vi "Organize Folders.vi"() -> ()   [LabVIEW 2024]
uses:
  <userlib>/_OpenG.lib/file/file.llb/Strip Path Extension - String__ogtk.vi
  <userlib>/_OpenG.lib/file/file.llb/openg_file.lvlib
panel:
  in  "clear filter":bool
  in  "move":bool
  in  "Series Data":i32(listbox)
  in  "Filter":string
  in  "Series Folders":i32(listbox)
  in  "Stop":bool
  in  "Top Folders":i32(listbox)
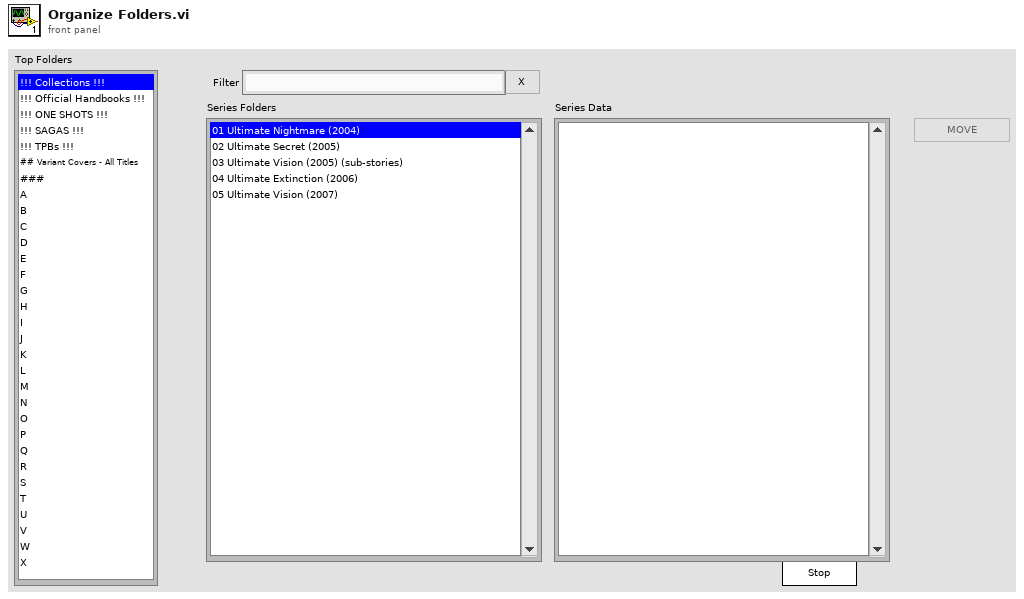
[diagram p1: front panel]
types:
  T1 = enum32{"Invalid", "Standard", "Closed", "Hidden", "Minimized", "Maximized"}
  T2 = enum32{"invalid app kind", "Development System", "Run Time System", "Student Edition", "Embedded LabVIEW", "Evaluation", "Custom"}
  T3 = enum8{"Enabled", "Disabled", "Disabled and Grayed Out"}
  T4 = cluster{"Core":cluster{"Current VI Reference":refnum<vi>, "Close Panel on Exit?":bool}, "parent path":path, "series folders":string[], "data.series path":path, "series data":string[], "old series path":path, "new series path":path}
  T5 = cluster{"Current VI Reference":refnum<vi>, "Close Panel on Exit?":bool}
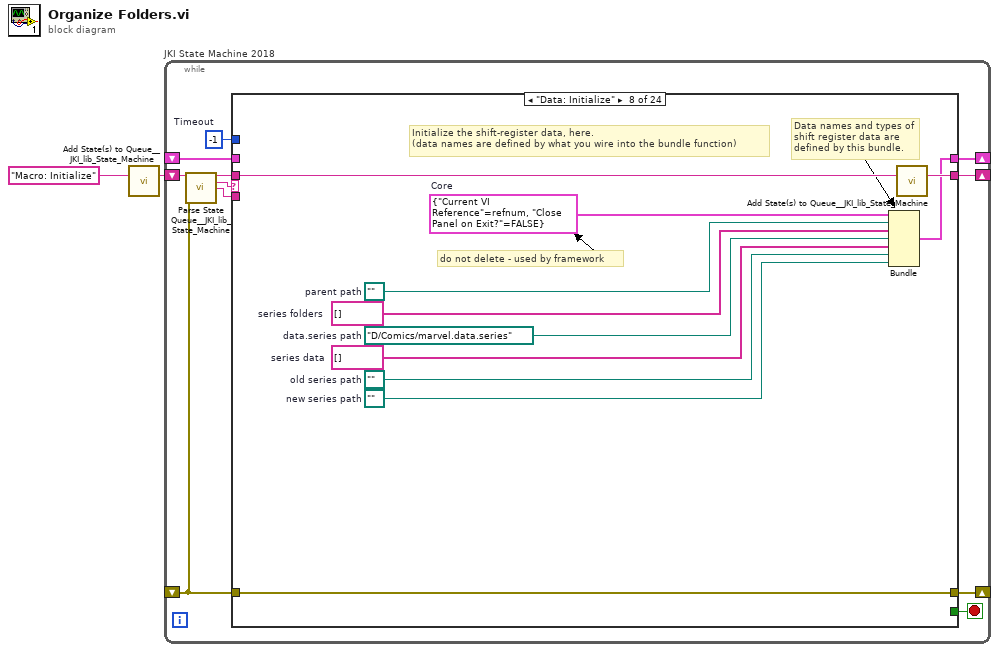
[diagram p0: block diagram]
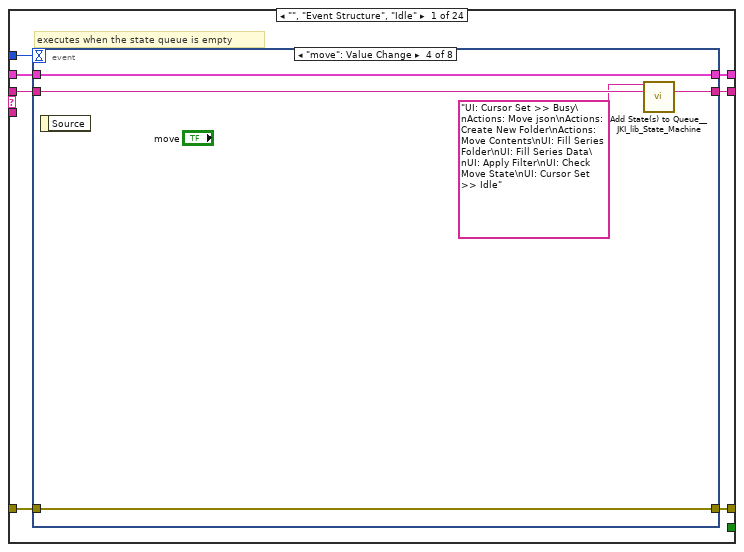
[diagram p2: hidden frame]
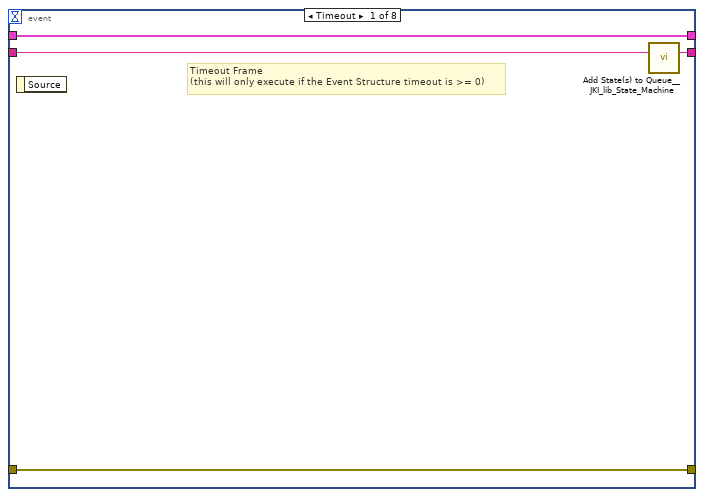
[diagram p3: hidden frame]
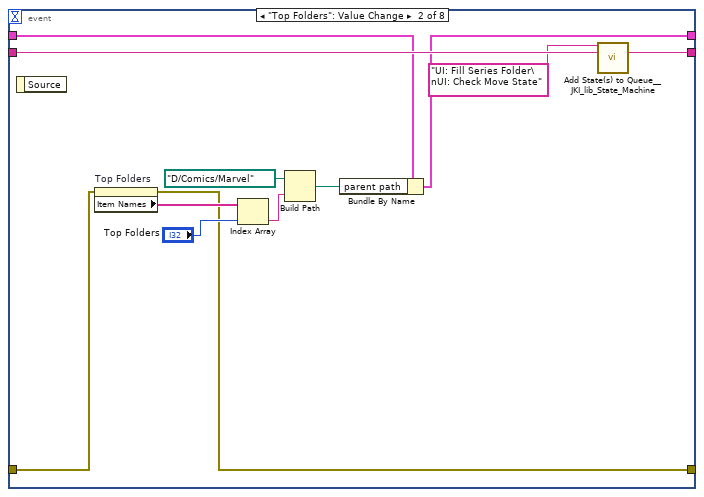
[diagram p4: hidden frame]
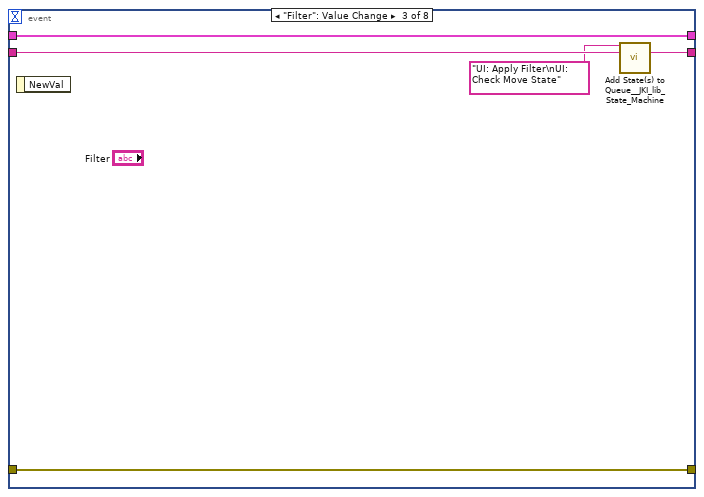
[diagram p5: hidden frame]
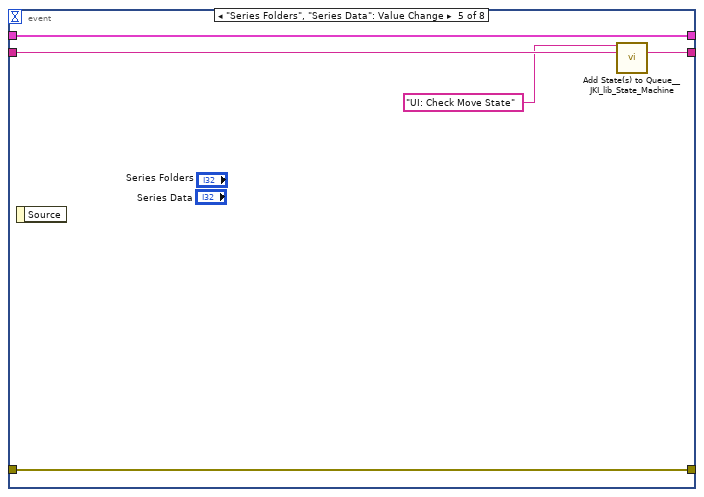
[diagram p6: hidden frame]
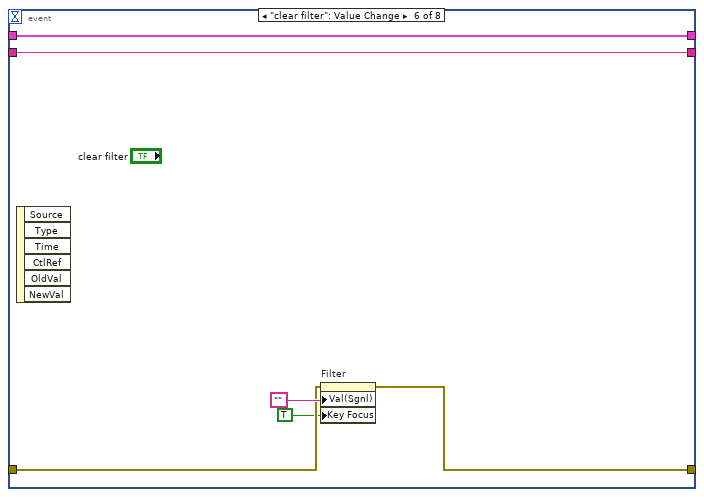
[diagram p7: hidden frame]
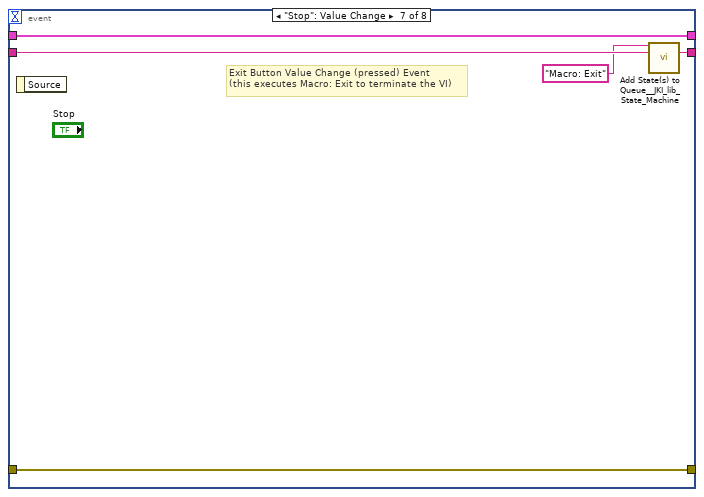
[diagram p8: hidden frame]
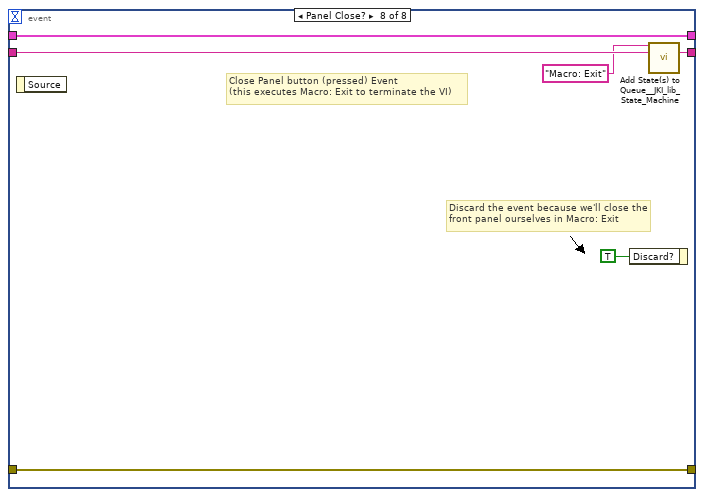
[diagram p9: hidden frame]
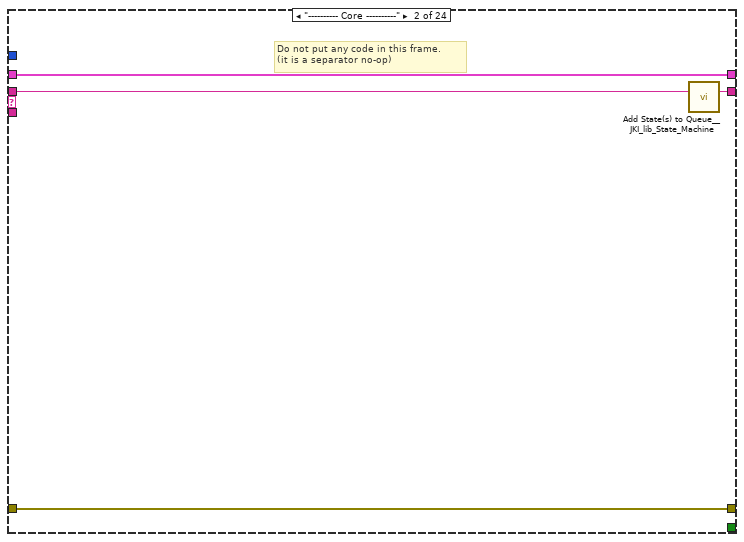
[diagram p10: hidden frame]
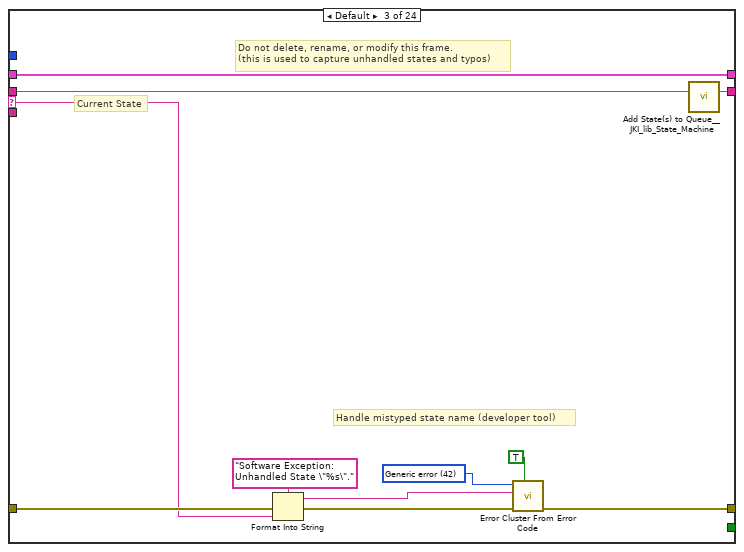
[diagram p11: hidden frame]
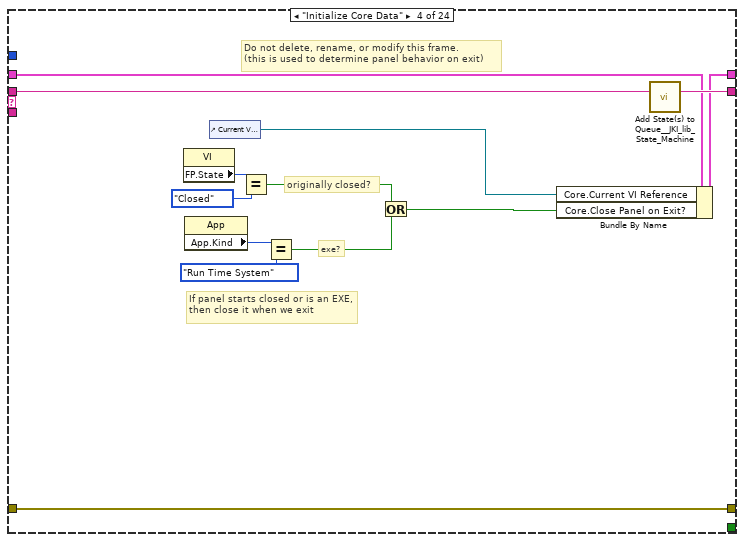
[diagram p12: hidden frame]
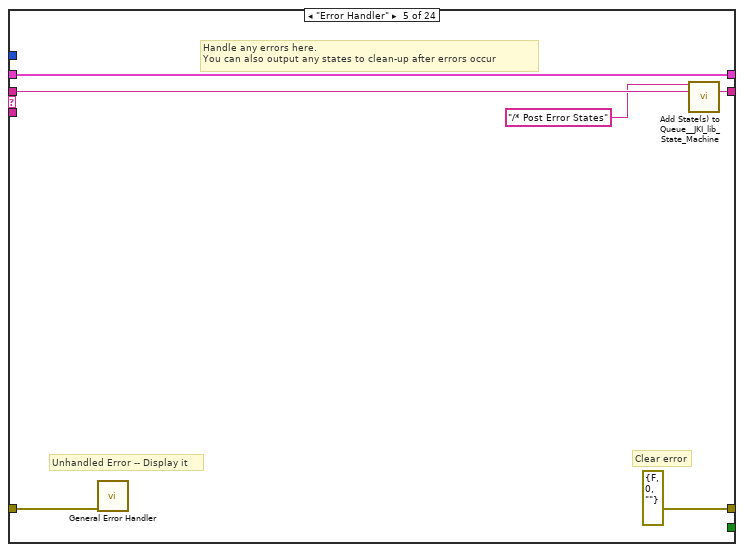
[diagram p13: hidden frame]
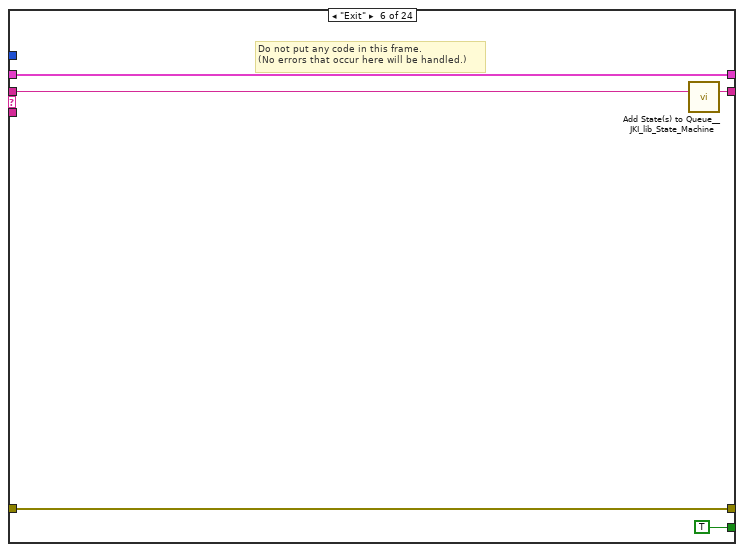
[diagram p14: hidden frame]
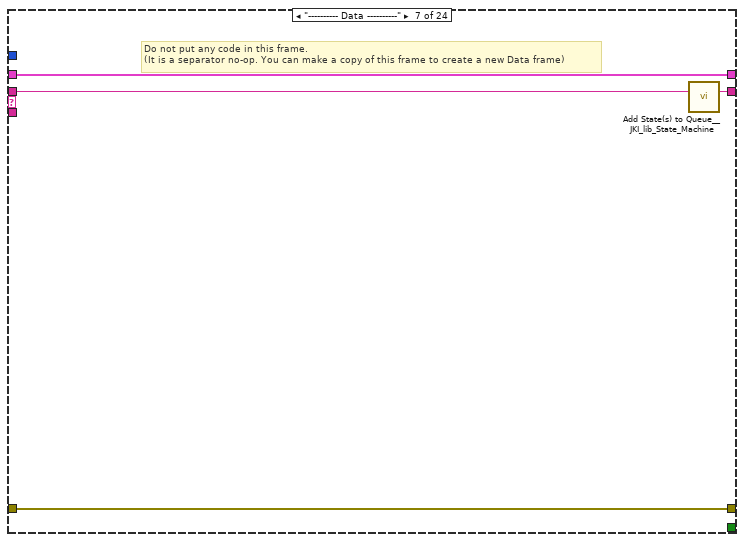
[diagram p15: hidden frame]
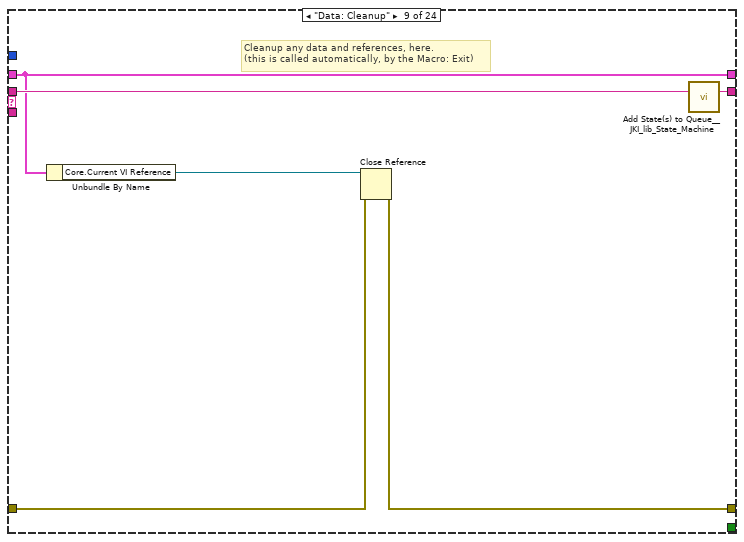
[diagram p16: hidden frame]
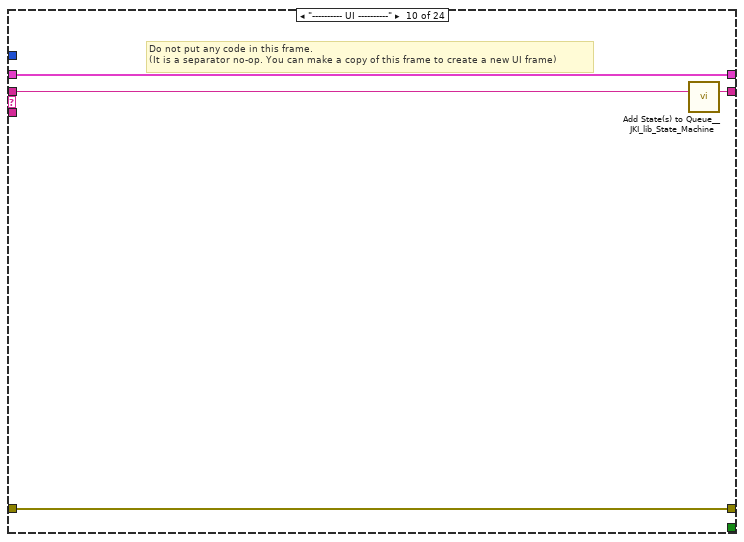
[diagram p17: hidden frame]
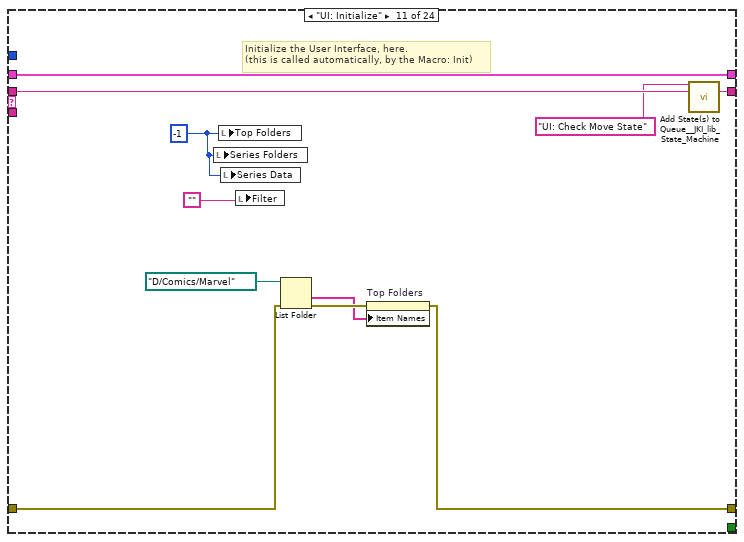
[diagram p18: hidden frame]
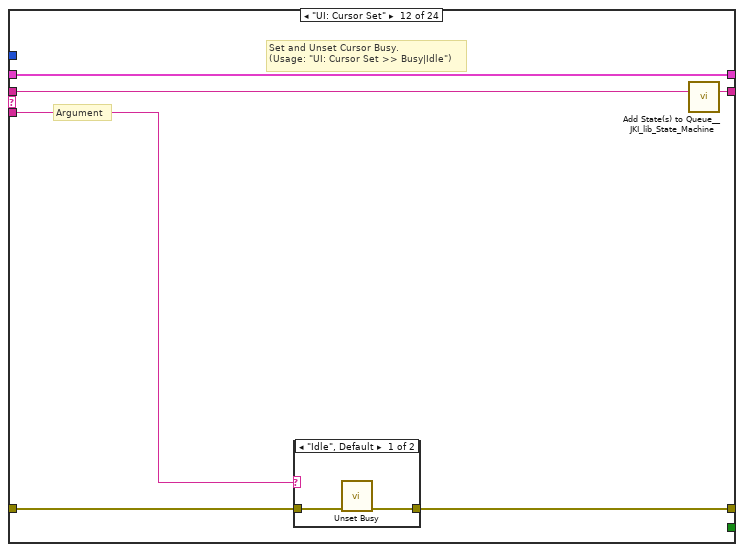
[diagram p19: hidden frame]
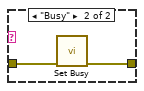
[diagram p20: hidden frame]
diagram:
  n1 = call <vilib>:"Add State(s) to Queue__JKI_lib_State_Machine.vi"("State(s) in (\"\")"="Macro: Initialize") -> ("States Out"=w2:string)  [unwired: 14 in]
  n2 = while "JKI State Machine 2018" {
    shift-right: [w6] -> _
    shift-left: _ -> [w5]
    shift-right: [w9] -> _
    shift-left: _ -> [w3]
    shift-right: [w8] -> _
    shift-left: w2 -> [w10]
    stop <- w7 stop-if-true
    w4 = -1  # Timeout
    n3 = call <vilib>:"Parse State Queue__JKI_lib_State_Machine.vi"("State Queue"=w10, "Error In (no error)"=w3) -> ("Remaining States"=w12:string, "Current State"=w13:string, "Arguments"=w11:string)  [unwired: 11 in]
    n4 = case shown="\"Data: Initialize\"" w13 {
      selector: w13 -> [_ _ w73 _ _ _ _ _ _ _ _ _ _ _ _ _ _ _ _ _ _ _ _ _]
      tunnel: w12 -> [w20 w72 w77 w96 w102 w107 w111 w122 w128 w132 w143 w149 w160 w234 w247 w259 w280 w285 w290 w300 w304 w323 w329 w337]
      tunnel: w11 -> [_ _ _ _ _ _ _ _ _ _ _ w144 w154 _ _ _ _ _ _ _ _ _ _ _]
      tunnel: w5 -> [w18 w69 w75 w89 w99 w105 w108 _ w123 w129 w141 w147 w156 w229 w242 w258 w281 w282 w287 w297 w301 w313 w327 w335]
      tunnel: [w17 w70 w79 w93 errorcluster {"status"=FALSE, "code"=0, "source"=""} ("error out") w104 w109 w119 w124 w130 w136 w145 w157 w230 w243 w252 w271 w283 w288 w298 w302 w316 w325 w333] -> w9
      tunnel: w3 -> [w16 w70 w78 w93 w98 w104 w109 w119 w125 w130 w137 w146 w158 w232 w245 w249 w270 w283 w288 w298 w302 w315 w324 w334]
      tunnel: [w19 w71 w76 w95 w101 w106 w110 w121 w127 w131 w142 w148 w159 w234 w247 w259 w280 w284 w289 w299 w303 w322 w328 w336] -> w8
      tunnel: [_ _ _ _ _ TRUE _ _ _ _ _ _ _ _ _ _ _ _ _ _ _ _ _ _] -> w7
      tunnel: [w15 w69 w75 w94 w99 w105 w108 w120 w123 w129 w141 w147 w156 w228 w241 w258 w281 w282 w287 w297 w301 w307 w327 w335] -> w6
      tunnel: w4 -> [w14 _ _ _ _ _ _ _ _ _ _ _ _ _ _ _ _ _ _ _ _ _ _ _]
      frame "", "Event Structure", "Idle" {
        # "executes when the state queue is empty"
        n5 = event shown="[3] \"move\": Value Change" {
          selector: _ -> [_ _ _ _ _ _ _ _]
          dyn-events: _ -> [_ _ _ _ _ _ _ _]
          timeout: w14 -> [_ _ _ _ _ _ _ _]
          tunnel: w20 -> [w24 w36 w40 w45 w50 w56 w62 w68]
          tunnel: [w23 w35 w39 w44 w49 w56 w61 w67] -> w19
          tunnel: w18 -> [w21 w29 w41 w46 w51 w57 w59 w65]
          tunnel: [w22 w25 w37 w42 w47 w52 w60 w66] -> w17
          tunnel: w16 -> [w22 w26 w37 w42 w47 w54 w60 w66]
          tunnel: [w21 w27 w41 w46 w51 w57 w59 w65] -> w15
          event Timeout {
            # "Timeout Frame\n(this will only execute if the Event Structure timeout is >= 0)"
            n6 = event-data() -> ()  [unwired: 1 in, 1 out]
            n7 = call <vilib>:"Add State(s) to Queue__JKI_lib_State_Machine.vi"("State(s) in (\"\")"=w24) -> ("States Out"=w23:string)  [unwired: 14 in]
          }
          event "Top Folders": Value Change {
            n8 = event-data() -> ()  [unwired: 1 in, 1 out]
            n9 = property on="Top Folders" class="LstBox (strict)"(error in=w26) -> (error out=w25:errorcluster, "Item Names"=w32:string[])  [unwired: 1 in, 1 out]
            n10 = Index Array(array=w32, index="Top Folders") -> (element=w30:string)
            n11 = Build Path(base path=path "D:/Comics/Marvel", name or relative path=w30) -> (appended path=w28:path)
            n12 = Bundle By Name(cluster=w29, "parent path"=w28) -> (w27:T4)
            n13 = call <vilib>:"Add State(s) to Queue__JKI_lib_State_Machine.vi"("State(s) in Front (\"\")"="UI: Fill Series Folder\nUI: Check Move State" ("State(s) in Front (\"\")"), "State(s) in (\"\")"=w36) -> ("States Out"=w35:string)  [unwired: 13 in]
          }
          event "Filter": Value Change {
            n14 = event-data() -> ()  [unwired: 1 in, 1 out]
            n15 = call <vilib>:"Add State(s) to Queue__JKI_lib_State_Machine.vi"("State(s) in Front (\"\")"="UI: Apply Filter\nUI: Check Move State" ("State(s) in Front (\"\")"), "State(s) in (\"\")"=w40) -> ("States Out"=w39:string)  [unwired: 13 in]
          }
          event "move": Value Change {
            n16 = event-data() -> ()  [unwired: 1 in, 1 out]
            n17 = call <vilib>:"Add State(s) to Queue__JKI_lib_State_Machine.vi"("State(s) in Front (\"\")"="UI: Cursor Set >> Busy\nActions: Move json\nActions: Create New Folder\nActions: Move Contents\nUI: Fill Series Folder\nUI: Fill Series Data\nUI: Apply Filter\nUI: Check Move State\nUI: Cursor Set >> Idle" ("State(s) in Front (\"\")"), "State(s) in (\"\")"=w45) -> ("States Out"=w44:string)  [unwired: 13 in]
          }
          event "Series Folders", "Series Data": Value Change {
            n18 = event-data() -> ()  [unwired: 1 in, 1 out]
            n19 = call <vilib>:"Add State(s) to Queue__JKI_lib_State_Machine.vi"("State(s) in Front (\"\")"="UI: Check Move State" ("State(s) in Front (\"\")"), "State(s) in (\"\")"=w50) -> ("States Out"=w49:string)  [unwired: 13 in]
          }
          event "clear filter": Value Change {
            n20 = event-data() -> ()  [unwired: 1 in, 6 out]
            n21 = property on="Filter" class="Str"(error in=w54, "Val(Sgnl)"="", "Key Focus"=TRUE) -> (error out=w52:errorcluster)  [unwired: 1 in, 1 out]
          }
          event "Stop": Value Change {
            # "Exit Button Value Change (pressed) Event\n(this executes Macro: Exit to terminate the VI)"
            n22 = event-data() -> ()  [unwired: 1 in, 1 out]
            n23 = call <vilib>:"Add State(s) to Queue__JKI_lib_State_Machine.vi"("State(s) in Front (\"\")"="Macro: Exit", "State(s) in (\"\")"=w62) -> ("States Out"=w61:string)  [unwired: 13 in]
          }
          event Panel Close? {
            # "Discard the event because we'll close the front panel ourselves in Macro: Exit"
            # "Close Panel button (pressed) Event\n(this executes Macro: Exit to terminate the VI)"
            n24 = event-data() -> ()  [unwired: 1 in, 1 out]
            n25 = event-data("Discard?"=TRUE) -> ()  [unwired: 1 in, 1 out]
            n26 = call <vilib>:"Add State(s) to Queue__JKI_lib_State_Machine.vi"("State(s) in Front (\"\")"="Macro: Exit", "State(s) in (\"\")"=w68) -> ("States Out"=w67:string)  [unwired: 13 in]
          }
        }
      }
      frame "---------- Core ----------" {
        # "Do not put any code in this frame.\n(it is a separator no-op)"
        n27 = call <vilib>:"Add State(s) to Queue__JKI_lib_State_Machine.vi"("State(s) in (\"\")"=w72) -> ("States Out"=w71:string)  [unwired: 14 in]
      }
      frame Default {
        w82 = 42 items=["No error", "Argument error", "Memory is full", "Out of zone", "End of file", "File already open", "Generic file I/O error", "File not found", "File permission error", "Disk is full", "Duplicate path", "Too many files open", "System feature not enabled", "Resource file not found", "Cannot add resource", "Resource not found", "Image not found", "Image memory error", "Pen does not exist", "Config type invalid", "Config token not found", "Config parse error", "Config memory error", "Bad external code format", "Bad external code offset", "External code not present", "Null window", "Destroy window error", "Null menu", "Print aborted", "Bad print record", "Print driver error", "Windows error during printing", "Memory error during printing", "Print dialog error", "Generic print error", "Invalid device refnum", "Device not found", "Device parameter error", "Device unit error", "Cannot open device", "Device call aborted", "Generic error", "Cancelled by user", "Object ID too low", "Object ID too high", "Object not in heap", "Unknown heap", "Unknown object (invalid DefProc)", "Unknown object (DefProc not in table)", "Message out of range", "Invalid (null) method", "Unknown message", "Manager call not supported", "Bad address", "Network operation in progress", "Network operation timed out", "Connection is busy", "Network attribute not supported", "Network error", "Address in use", "System out of memory", "Connection aborted", "Connection refused", "Not connected", "Already connected", "Connection closed", "Initialization error (interapplication manager)", "Bad occurrence", "Wait on unbound occurrence handler", "Occurrence queue overflow", "Datalog type conflict", "Unused", "Unrecognized type (interapplication manager)", "Memory corrupt", "Failed to make temporary DLL", "Old CIN version", "Drag socket not found", "Failed to load drop-object", "Failed to register OLE object", "Failed to release OLE object", "Format specifier type mismatch", "Unknown format specifier", "Too few format specifiers", "Too many format specifiers", "Scan failed", "Newer CIN version", "Error converting to variant", "Runtime menu error", "Password tampered", "Variant attribute not found", "Incompatible variant data type", "Event data is not available", "Event Store is not present", "Occurrence is not found", "Event Queue is not created", "Event info is not available", "Refnum passed is NULL", "Error retrieving Class GUID", "Error retrieving CoClass GUID", "Error retrieving TypeLib GUID.", "Bad built application magic bytes.", "Specific driver is different from the specific driver associated with the Logical Name.", "There is no session opened to the class driver.", "Max Error", "MAX - Error with config objects", "MAX - Error loading configuration", "MAX - Group not supported"]
        # "Current State"
        # "Do not delete, rename, or modify this frame.\n(this is used to capture unhandled states and typos)"
        # "Handle mistyped state name (developer tool)"
        n28 = Format Into String(format string="Software Exception: Unhandled State \"%s\"." ("message"), error in=w78, w73) -> (resulting string=w81:string, error out=w80:errorcluster)  [unwired: 1 in]
        n29 = call <vilib>:"Error Cluster From Error Code.vi"("show call chain? (False)"=TRUE, "error in (no error)"=w80, "error message (\"\")"=w81, "error code (0)"=w82) -> ("error out"=w79:errorcluster)  [unwired: 5 in]
        n30 = call <vilib>:"Add State(s) to Queue__JKI_lib_State_Machine.vi"("State(s) in (\"\")"=w77) -> ("States Out"=w76:string)  [unwired: 14 in]
      }
      frame "Initialize Core Data" {
        # "Do not delete, rename, or modify this frame.\n(this is used to determine panel behavior on exit)"
        # "originally closed?"
        # "exe?"
        # "If panel starts closed or is an EXE, then close it when we exit"
        n31 = property class="VI"() -> ("FP.State"=w86:T1)  [unwired: 2 in, 2 out]
        n32 = property class="App"() -> ("App.Kind"=w92:T2)  [unwired: 2 in, 2 out]
        n33 = control-ref of="Current VI Reference"() -> (w87:refnum<vi>)
        n34 = Equal?(x=w86, y=T1."Closed" ("Front Panel Window:State")) -> (x = y?=w84:bool)
        n35 = Equal?(x=w92, y=T2."Run Time System" ("Application:Kind")) -> (x = y?=w90:bool)
        n36 = Or(x=w84, y=w90) -> (x .or. y?=w88:bool)
        n37 = Bundle By Name(cluster=w89, "Core.Current VI Reference"=w87, "Core.Close Panel on Exit?"=w88) -> (w94:T4)
        n38 = call <vilib>:"Add State(s) to Queue__JKI_lib_State_Machine.vi"("State(s) in (\"\")"=w96) -> ("States Out"=w95:string)  [unwired: 14 in]
      }
      frame "Error Handler" {
        # "Unhandled Error -- Display it"
        # "Handle any errors here.\nYou can also output any states to clean-up after errors occur"
        # "Clear error"
        n39 = call <vilib>:"General Error Handler.vi"("error in (no error)"=w98) -> ()  [unwired: 10 in, 5 out]
        n40 = call <vilib>:"Add State(s) to Queue__JKI_lib_State_Machine.vi"("State(s) in Front (\"\")"="/* Post Error States", "State(s) in (\"\")"=w102) -> ("States Out"=w101:string)  [unwired: 13 in]
      }
      frame "Exit" {
        # "Do not put any code in this frame.\n(No errors that occur here will be handled.)"
        n41 = call <vilib>:"Add State(s) to Queue__JKI_lib_State_Machine.vi"("State(s) in (\"\")"=w107) -> ("States Out"=w106:string)  [unwired: 14 in]
      }
      frame "---------- Data ----------" {
        # "Do not put any code in this frame.\n(It is a separator no-op. You can make a copy of this frame to create a new Data frame)"
        n42 = call <vilib>:"Add State(s) to Queue__JKI_lib_State_Machine.vi"("State(s) in (\"\")"=w111) -> ("States Out"=w110:string)  [unwired: 14 in]
      }
      frame "Data: Initialize" {
        w112 = path ""  # new series path
        w113 = path ""  # old series path
        w114 = string[] []  # series data
        w115 = path "D:/Comics/marvel.data.series"  # data.series path
        w116 = T5 {"Current VI Reference"=refnum, "Close Panel on Exit?"=FALSE}  # Core
        w118 = path ""  # parent path
        w117 = string[] []  # series folders
        # "do not delete - used by framework"
        # "Data names and types of shift register data are defined by this bundle."
        # "Initialize the shift-register data, here.\n(data names are defined by what you wire into the bundle function)"
        n43 = Bundle("Core"=w116, "parent path"=w118, "series folders"=w117, "data.series path"=w115, "series data"=w114, "old series path"=w113, "new series path"=w112) -> (w120:T4)  [unwired: 1 in]
        n44 = call <vilib>:"Add State(s) to Queue__JKI_lib_State_Machine.vi"("State(s) in (\"\")"=w122) -> ("States Out"=w121:string)  [unwired: 14 in]
      }
      frame "Data: Cleanup" {
        # "Cleanup any data and references, here.\n(this is called automatically, by the Macro: Exit)"
        n45 = Unbundle By Name(w123) -> ("Core.Current VI Reference"=w126:refnum<vi>)
        n46 = Close Reference(reference=w126, error in (no error)=w125) -> (error out=w124:errorcluster)
        n47 = call <vilib>:"Add State(s) to Queue__JKI_lib_State_Machine.vi"("State(s) in (\"\")"=w128) -> ("States Out"=w127:string)  [unwired: 14 in]
      }
      frame "---------- UI ----------" {
        # "Do not put any code in this frame.\n(It is a separator no-op. You can make a copy of this frame to create a new UI frame)"
        n48 = call <vilib>:"Add State(s) to Queue__JKI_lib_State_Machine.vi"("State(s) in (\"\")"=w132) -> ("States Out"=w131:string)  [unwired: 14 in]
      }
      frame "UI: Initialize" {
        w135 = -1 ("Top Folders")
        # "Initialize the User Interface, here.\n(this is called automatically, by the Macro: Init)"
        n49 = local write "Series Folders"(w135) -> ()
        n50 = local write "Top Folders"(w135) -> ()
        n51 = local write "Series Data"(w135) -> ()
        n52 = local write "Filter"("") -> ()
        n53 = List Folder(path=path "D:/Comics/Marvel", error in=w137) -> (folder names=w139:string[], error out=w140:errorcluster)  [unwired: 2 in, 2 out]
        n54 = property on="Top Folders" class="LstBox (strict)"(error in=w140, "Item Names"=w139) -> (error out=w136:errorcluster)  [unwired: 1 in, 1 out]
        n55 = call <vilib>:"Add State(s) to Queue__JKI_lib_State_Machine.vi"("State(s) in Front (\"\")"="UI: Check Move State" ("State(s) in Front (\"\")"), "State(s) in (\"\")"=w143) -> ("States Out"=w142:string)  [unwired: 13 in]
      }
      frame "UI: Cursor Set" {
        # "Argument"
        # "Set and Unset Cursor Busy.\n(Usage: \"UI: Cursor Set >> Busy|Idle\")"
        n56 = case shown="\"Idle\", Default" w144 {
          tunnel: w146 -> [w151 w153]
          tunnel: [w150 w152] -> w145
          frame "Idle", Default {
            n57 = call <vilib>:"Unset Busy.vi"("error in (no error)"=w151) -> ("error out"=w150:errorcluster)  [unwired: 10 in]
          }
          frame "Busy" {
            n58 = call <vilib>:"Set Busy.vi"("error in (no error)"=w153) -> ("error out"=w152:errorcluster)  [unwired: 9 in, 1 out]
          }
        }
        n59 = call <vilib>:"Add State(s) to Queue__JKI_lib_State_Machine.vi"("State(s) in (\"\")"=w149) -> ("States Out"=w148:string)  [unwired: 14 in]
      }
      frame "UI: Front Panel State" {
        # "Argument"
        # "Set Front Panel Open or Closed\n(Usage: \"UI: Front Panel State >> Open|Close\")"
        n60 = Unbundle By Name(w156) -> ("Core.Current VI Reference"=w155:refnum<vi>)
        n61 = case shown="\"Minimize\", \"Minimized\"" w154 {
          tunnel: w158 -> [w166 w181 w192 w205 w218]
          tunnel: [w168 w182 w194 w207 w220] -> w157
          tunnel: w155 -> [w167 w179 w193 w206 w219]
          frame "Open", "Standard", Default {
            w161 = T1."Standard" ("State")
            n62 = property class="VI"(reference=w167, error in=w166) -> (reference out=w164:refnum<vi>, error out=w165:errorcluster, "FP.State"=w163:T1)
            n63 = Not Equal?(x=w163, y=w161) -> (x != y?=w162:bool)
            n64 = case shown="True" w162 {
              tunnel: [w172 w174] -> w168
              tunnel: w165 -> [w171 w174]
              tunnel: w164 -> [w170 _]
              tunnel: w161 -> [w169 _]
              frame True {
                n65 = invoke class="VI" method="FP.Open"(reference=w170, error in=w171, "Activate"=TRUE, "State"=w169) -> (error out=w172:errorcluster)  [unwired: 1 in, 4 out]
              }
              frame False {
              }
            }
          }
          frame "Close", "Closed" {
            n66 = property class="VI"(reference=w179, error in=w181) -> (reference out=w178:refnum<vi>, error out=w180:errorcluster, "FP.State"=w176:T1)
            n67 = Not Equal?(x=w176, y=T1."Closed" ("Front Panel Window:State")) -> (x != y?=w175:bool)
            n68 = case shown="True" w175 {
              tunnel: [w183 w186] -> w182
              tunnel: w180 -> [w183 w185]
              tunnel: w178 -> [_ w184]
              frame False {
              }
              frame True {
                n69 = invoke class="VI" method="FP.Close"(reference=w184, error in=w185) -> (error out=w186:errorcluster)  [unwired: 1 in, 2 out]
              }
            }
          }
          frame "Hidden", "Hide" {
            w187 = T1."Hidden" ("State")
            n70 = property class="VI"(reference=w193, error in=w192) -> (reference out=w190:refnum<vi>, error out=w191:errorcluster, "FP.State"=w189:T1)
            n71 = Not Equal?(x=w189, y=w187) -> (x != y?=w188:bool)
            n72 = case shown="True" w188 {
              tunnel: [w198 w199] -> w194
              tunnel: w191 -> [w197 w199]
              tunnel: w190 -> [w196 _]
              tunnel: w187 -> [w195 _]
              frame True {
                n73 = invoke class="VI" method="FP.Open"(reference=w196, error in=w197, "State"=w195) -> (error out=w198:errorcluster)  [unwired: 2 in, 4 out]
              }
              frame False {
              }
            }
          }
          frame "Minimize", "Minimized" {
            w200 = T1."Minimized" ("State")
            n74 = property class="VI"(reference=w206, error in=w205) -> (reference out=w203:refnum<vi>, error out=w204:errorcluster, "FP.State"=w202:T1)
            n75 = Not Equal?(x=w202, y=w200) -> (x != y?=w201:bool)
            n76 = case shown="True" w201 {
              tunnel: [w211 w212] -> w207
              tunnel: w204 -> [w210 w212]
              tunnel: w203 -> [w209 _]
              tunnel: w200 -> [w208 _]
              frame True {
                n77 = invoke class="VI" method="FP.Open"(reference=w209, error in=w210, "State"=w208) -> (error out=w211:errorcluster)  [unwired: 2 in, 4 out]
              }
              frame False {
              }
            }
          }
          frame "Maximize", "Maximized" {
            w213 = T1."Maximized" ("State")
            n78 = property class="VI"(reference=w219, error in=w218) -> (reference out=w216:refnum<vi>, error out=w217:errorcluster, "FP.State"=w215:T1)
            n79 = Not Equal?(x=w215, y=w213) -> (x != y?=w214:bool)
            n80 = case shown="True" w214 {
              tunnel: [w224 w225] -> w220
              tunnel: w217 -> [w223 w225]
              tunnel: w216 -> [w222 _]
              tunnel: w213 -> [w221 _]
              frame True {
                n81 = invoke class="VI" method="FP.Open"(reference=w222, error in=w223, "State"=w221) -> (error out=w224:errorcluster)  [unwired: 2 in, 4 out]
              }
              frame False {
              }
            }
          }
        }
        n82 = call <vilib>:"Add State(s) to Queue__JKI_lib_State_Machine.vi"("State(s) in (\"\")"=w160) -> ("States Out"=w159:string)  [unwired: 14 in]
      }
      frame "UI: Fill Series Folder" {
        n83 = Unbundle By Name(w229) -> ("parent path"=w233:path)
        n84 = List Folder(path=w233, error in=w232) -> (folder names=w227:string[], error out=w231:errorcluster)  [unwired: 2 in, 2 out]
        n85 = for {
          tunnel: w227 -> [w236] mode=indexing
          tunnel: [w236] -> w226 mode=indexing if=w235
          n86 = Match Pattern(string=w236, regular expression="\\[") -> (offset past match=w237:i32)  [unwired: 1 in, 3 out]
          n87 = Less Than 0?(x=w237) -> (x < 0?=w235:bool)
        }
        n88 = property on="Series Folders" class="LstBox (strict)"(error in=w231, "Item Names"=w226) -> (error out=w230:errorcluster)  [unwired: 1 in, 1 out]
        n89 = Bundle By Name(cluster=w229, "series folders"=w226) -> (w228:T4)
      }
      frame "UI: Fill Series Data" {
        n90 = Unbundle By Name(w242) -> ("data.series path"=w246:path)
        n91 = List Folder(path=w246, error in=w245) -> (filenames=w240:string[], error out=w244:errorcluster)  [unwired: 2 in, 2 out]
        n92 = property on="Series Data" class="LstBox (strict)"(error in=w244, "Item Names"=w240, "FocusRow"=0 ("Top Row")) -> (error out=w243:errorcluster)  [unwired: 1 in, 1 out]
        n93 = Bundle By Name(cluster=w242, "series data"=w240) -> (w241:T4)
      }
      frame "UI: Apply Filter" {
        n94 = local read "Filter"() -> (w254:string)
        n95 = Unbundle By Name(w258) -> ("series folders"=w257:string[], "series data"=w253:string[])
        n96 = To Lower Case(string=w254) -> (all lower case string=w248:string)
        n97 = for {
          tunnel: w248 -> [w269]
          tunnel: w257 -> [w267] mode=indexing
          tunnel: [w267] -> w256 mode=indexing if=w266
          n98 = To Lower Case(string=w267) -> (all lower case string=w265:string)
          n99 = Match Pattern(string=w265, regular expression=w269) -> (offset past match=w268:i32)  [unwired: 1 in, 3 out]
          n100 = Greater Or Equal To 0?(x=w268) -> (x >= 0?=w266:bool)
        }
        n101 = for {
          tunnel: w248 -> [w264]
          tunnel: w253 -> [w262] mode=indexing
          tunnel: [w262] -> w255 mode=indexing if=w261
          n102 = To Lower Case(string=w262) -> (all lower case string=w260:string)
          n103 = Match Pattern(string=w260, regular expression=w264) -> (offset past match=w263:i32)  [unwired: 1 in, 3 out]
          n104 = Greater Or Equal To 0?(x=w263) -> (x >= 0?=w261:bool)
        }
        n105 = property on="Series Folders" class="LstBox (strict)"(error in=w249, "Item Names"=w256) -> (error out=w250:errorcluster)  [unwired: 1 in, 1 out]
        n106 = property on="Series Data" class="LstBox (strict)"(error in=w249, "Item Names"=w255) -> (error out=w251:errorcluster)  [unwired: 1 in, 1 out]
        n107 = Merge Errors(w250, w251, w249) -> (w252:errorcluster)
      }
      frame "UI: Check Move State" {
        n108 = local read "Series Data"() -> (w279:i32)
        n109 = local read "Series Folders"() -> (w278:i32)
        n110 = Less Than 0?(x=w279) -> (x < 0?=w277:bool)
        n111 = Less Than 0?(x=w278) -> (x < 0?=w276:bool)
        n112 = Or(x=w277, y=w276) -> (x .or. y?=w275:bool)
        n113 = Select(t=T3."Disabled and Grayed Out", s=w275, f=T3."Enabled" ("Disabled")) -> (s? t:f=w273:T3)
        n114 = property on="move" class="Bool"(error in=w270, "DisabledEnum"=w273) -> (error out=w271:errorcluster)  [unwired: 1 in, 1 out]
      }
      frame "---------- Macro ----------" {
        # "Do not put any code in this frame.\n(It is a separator no-op. You can make a copy of this frame to create a new Macro frame)"
        n115 = call <vilib>:"Add State(s) to Queue__JKI_lib_State_Machine.vi"("State(s) in (\"\")"=w285) -> ("States Out"=w284:string)  [unwired: 14 in]
      }
      frame "Macro: Initialize" {
        w286 = "Data: Initialize\nInitialize Core Data\nUI: Initialize\nUI: Front Panel State >> Open\nUI: Fill Series Data "  # Data: Initialize Initialize Core Data UI: Initialize UI: Front Panel State >> Open UI: Fill Series Data
        # "Initialization Macro\n(This is called once, when the VI starts)"
        n116 = call <vilib>:"Add State(s) to Queue__JKI_lib_State_Machine.vi"("State(s) in Front (\"\")"=w286, "State(s) in (\"\")"=w290) -> ("States Out"=w289:string)  [unwired: 13 in]
      }
      frame "Macro: Exit" {
        # "Exit Macro\n(This is called once, when the VI exits)"
        n117 = Unbundle By Name(w297) -> ("Core.Close Panel on Exit?"=w296:bool)
        n118 = Select(t="UI: Front Panel State >> Close", s=w296, f="") -> (s? t:f=w293:string)
        n119 = call <vilib>:"Add State(s) to Queue__JKI_lib_State_Machine.vi"("State(s) in (\"\")"=w293, "State(s) at Back (\"\")"="Data: Cleanup\nExit") -> ("States Out"=w291:string)  [unwired: 13 in]
        n120 = call <vilib>:"Add State(s) to Queue__JKI_lib_State_Machine.vi"("State(s) in Front (\"\")"=w291, "State(s) in (\"\")"=w300) -> ("States Out"=w299:string)  [unwired: 13 in]
      }
      frame "---------- Actions ----------" {
        # "Template Separator\n(You can make a copy of, or modify, this frame)"
        n121 = call <vilib>:"Add State(s) to Queue__JKI_lib_State_Machine.vi"("State(s) in (\"\")"=w304) -> ("States Out"=w303:string)  [unwired: 14 in]
      }
      frame "Actions: Move json" {
        n122 = local read "Series Folders"() -> (w306:i32)
        n123 = Unbundle By Name(w313) -> ("parent path"=w309:path, "data.series path"=w318:path)
        n124 = local read "Series Data"() -> (w305:i32)
        n125 = property on="Series Folders" class="LstBox (strict)"() -> ("Item Names"=w321:string[])  [unwired: 2 in, 2 out]
        n126 = property on="Series Data" class="LstBox (strict)"() -> ("Item Names"=w320:string[])  [unwired: 2 in, 2 out]
        n127 = Index Array(array=w321, index=w306) -> (element=w319:string)
        n128 = Index Array(array=w320, index=w305) -> (element=w311:string)
        n129 = Build Path(base path=w318, name or relative path=w311) -> (appended path=w314:path)
        n130 = call-poly <userlib>:"Strip Path Extension__ogtk.vi"("path"=w311) -> ("root"=w310:string)  [unwired: 1 out]
        n131 = Build Path(base path=w309, name or relative path=w319) -> (appended path=w312:path)
        n132 = Build Path(base path=w312, name or relative path=w311) -> (appended path=w317:path)
        n133 = Build Path(base path=w309, name or relative path=w310) -> (appended path=w308:path)
        n134 = Move(source path=w314, error in=w315, 10:w317) -> (error out=w316:errorcluster)  [unwired: 2 in, 2 out]
        n135 = Bundle By Name(cluster=w313, "old series path"=w312, "new series path"=w308) -> (w307:T4)
        n136 = call <vilib>:"Add State(s) to Queue__JKI_lib_State_Machine.vi"("State(s) in (\"\")"=w323) -> ("States Out"=w322:string)  [unwired: 14 in]
      }
      frame "Actions: Create New Folder" {
        n137 = Unbundle By Name(w327) -> ("new series path"=w326:path)
        n138 = Create Folder(path (use dialog)=w326, error in=w324) -> (error out=w325:errorcluster)  [unwired: 1 in, 2 out]
        n139 = call <vilib>:"Add State(s) to Queue__JKI_lib_State_Machine.vi"("State(s) in (\"\")"=w329) -> ("States Out"=w328:string)  [unwired: 14 in]
      }
      frame "Actions: Move Contents" {
        w330 = TRUE  # Delete Source Dir?
        n140 = Unbundle By Name(w335) -> ("new series path"=w332:path, "old series path"=w331:path)
        n141 = call "MoveFilesRecursively.vi"("Delete Source Dir?"=w330, "error in"=w334, "Dest Path"=w332, "Source Path"=w331) -> ("error out"=w333:errorcluster)  [unwired: 7 in]
        n142 = call <vilib>:"Add State(s) to Queue__JKI_lib_State_Machine.vi"("State(s) in (\"\")"=w337) -> ("States Out"=w336:string)  [unwired: 14 in]
      }
    }
  }
